vi "1_VNA_direct_spectrum_field_sweep_TEMPEATURE_(2D_PNA_m_Field_Direct_spec_RHUL).vi"() -> ()   [LabVIEW 2013]
uses:
  <vilib>/Analysis/baseanly.llb/Mean (DBL).vi
  <vilib>/Analysis/NI_AALBase.lvlib
panel:
  in  "Boolean 2":bool
  in  "?":enum32{"VNA"}(tab)
  out "Numeric":i32
  in  "Measurement \nper temperature":i32=3 caption="Delay Time (s)"
  out "Paused":bool
  in  "Boolean":bool
  in  "Delay Time (s)":dbl=3.0
  in  "?":enum32{"VNA"}(tab)
  in  "VNA Power dBm":dbl=-30.0 caption="VNA Power (dBm)" format="%#.3f"
  in  "Center Freq (Hz)":dbl=9000000000.0 caption="Center Freq (Hz):" format="%#.6p"
  in  "Span Freq:":dbl=14000000000.0 caption="Span Freq (Hz)" format="%#.3p"
  in  "Bandwidth:":dbl=10.0 caption="Bandwidth (1 to 1e6 Hz)" format="%#.3f"
  in  "Points:":i32=201 caption="Points"
  out "Phase (now)":dbl[](graph)
  out "Amplitude (now)":dbl[](graph)
  in  "Phase delay (ns)":dbl=53.6 format="%#_8g"
  in  "Offset (rad)":dbl
  out "Temperature sorted":dbl[](array[numeric])
  out "Phase Background Corrected":dbl[][](graph)
  out "Amplitude Background Corrected":dbl[][](graph)
  out "Phase Raw":dbl[][](graph)
  out "Amplitude Raw":dbl[][](graph)
  out "XY Graph":cluster{dbl[], dbl[]}(graph)
  out "Temp_start":dbl=2.0 format="%#_13g"
  out "Temp_end":dbl=16.0 format="%#_13g"
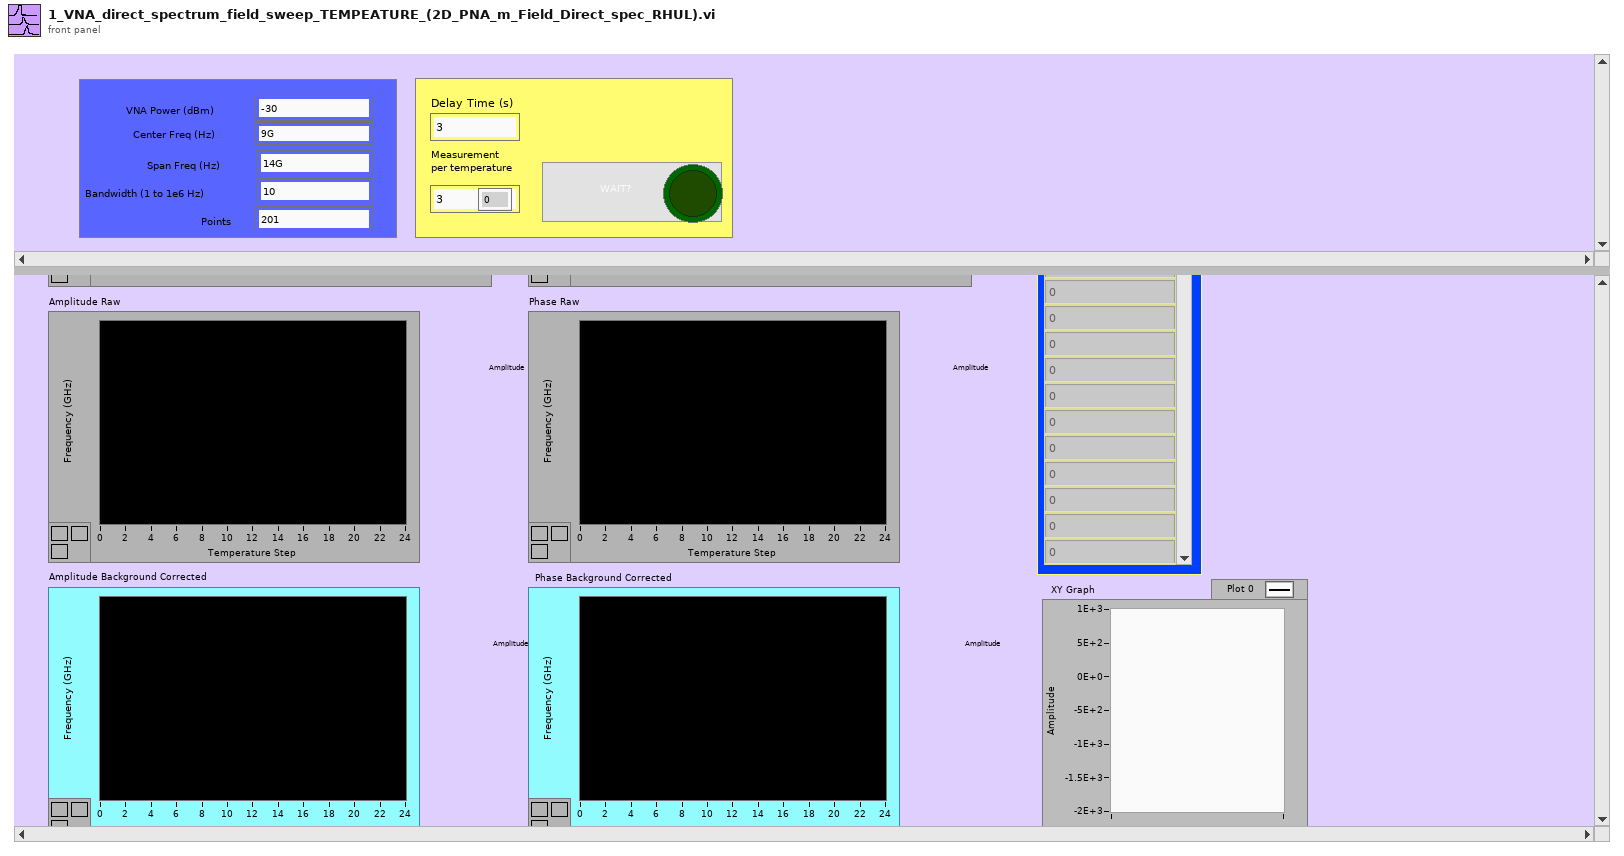
[diagram p1: front panel]
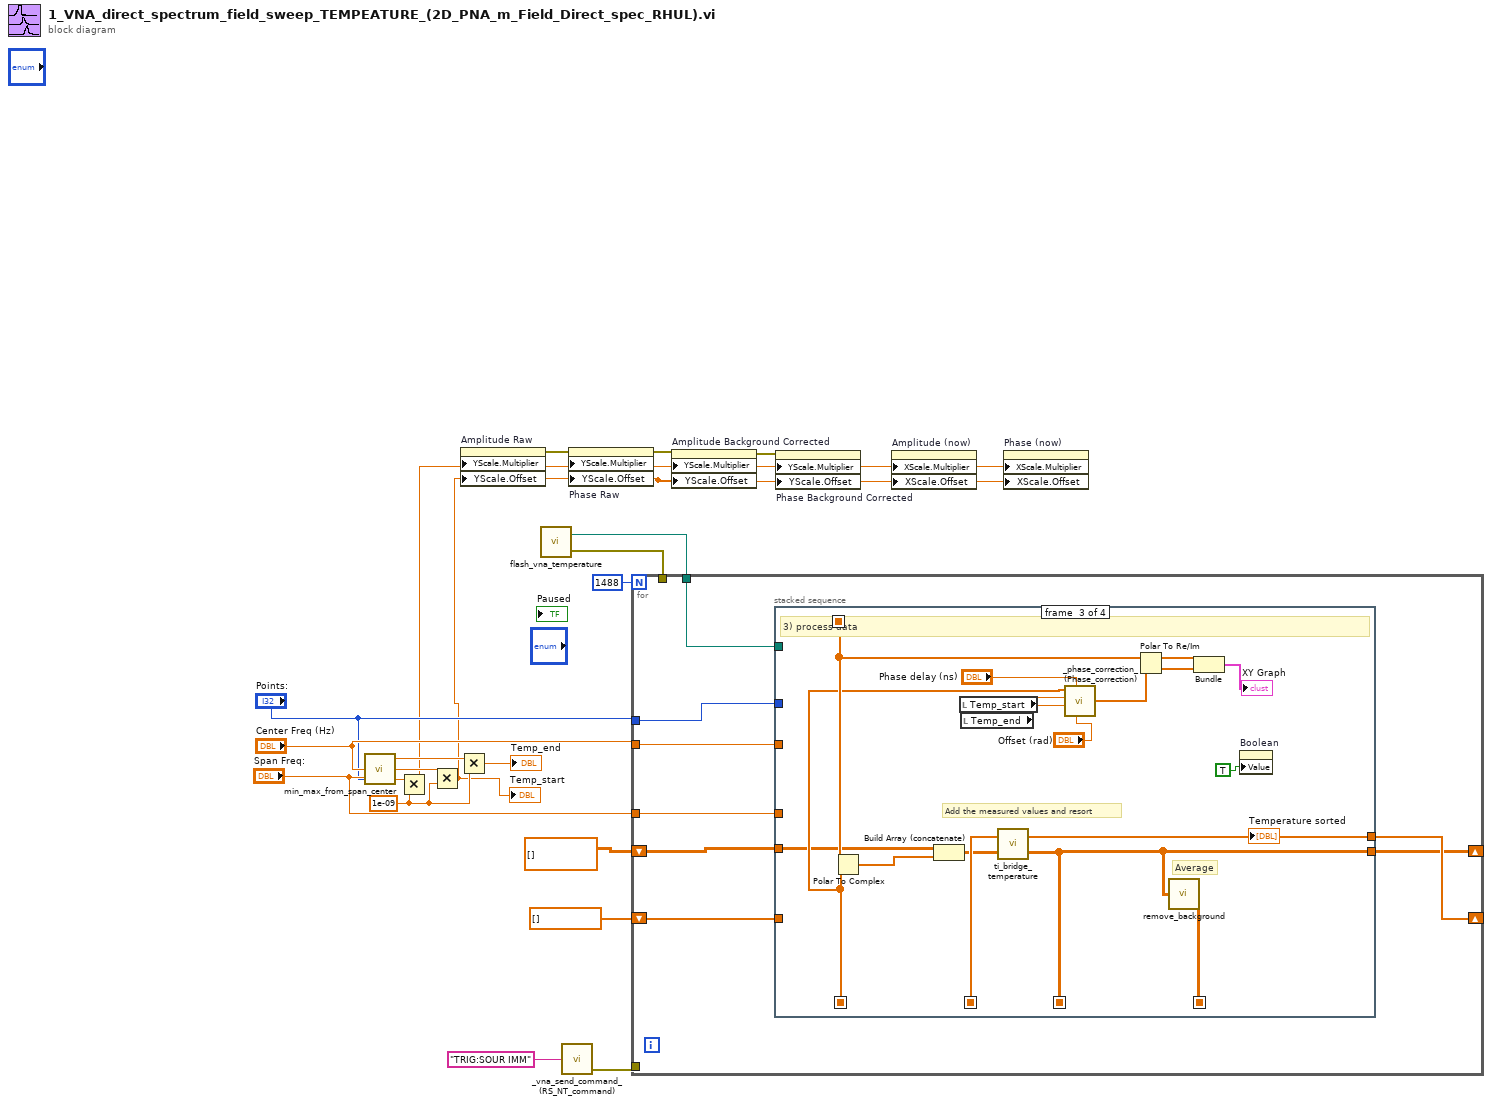
[diagram p0: block diagram]
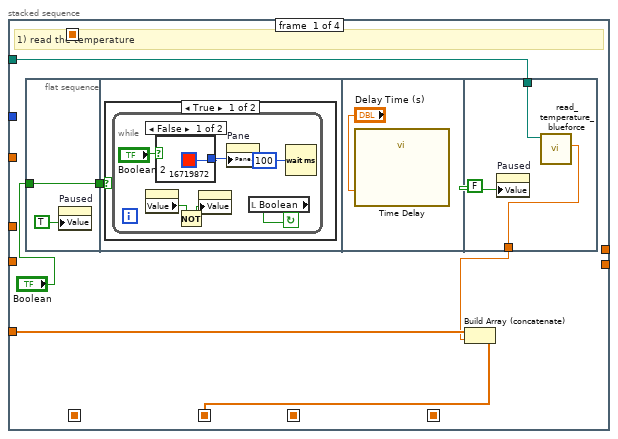
[diagram p2: hidden frame]
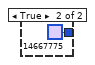
[diagram p3: hidden frame]
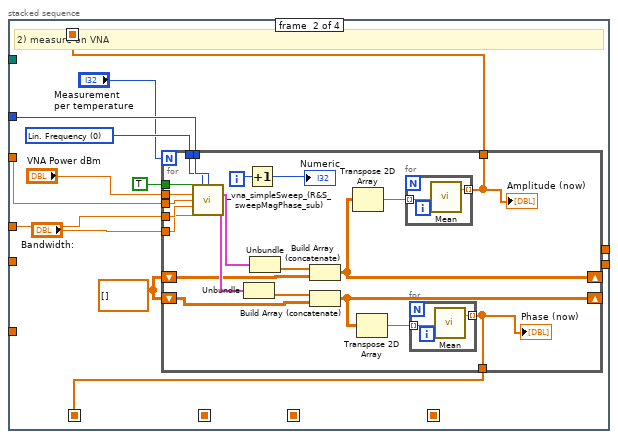
[diagram p5: hidden frame]
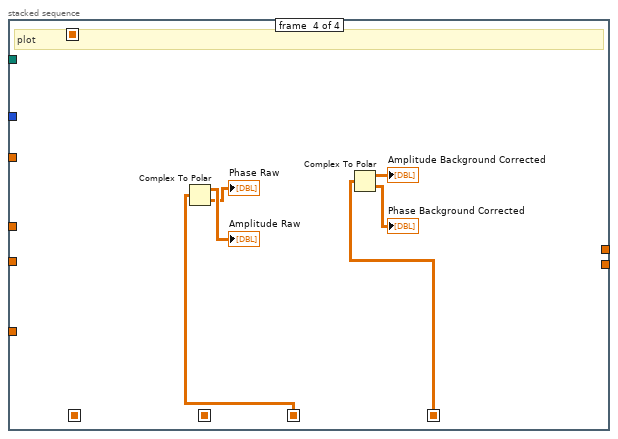
[diagram p6: hidden frame]
diagram:
  w13 = 1e-09
  n1 = call "min_max_from_span_center.vi"("No Points"="Points:", "Mid Point"="Center Freq (Hz)", "Span"="Span Freq:") -> ("Step"=w15:dbl, "Start"=w14:dbl, "End"=w18:dbl)
  n2 = Multiply(x=w15, y=w13) -> (x*y=w4:dbl)
  n3 = Multiply(x=w14, y=w13) -> (x*y=w3:dbl)
  "Temp_start" <- w3
  n4 = Multiply(x=w18, y=w13) -> (x*y=→"Temp_end":dbl)
  n5 = property on="Amplitude Raw" class="IntGraph (strict)"("YScale.Multiplier"=w4, "YScale.Offset"=w3) -> (error out=w7:errorcluster)  [unwired: 2 in, 1 out]
  n6 = call "flash_vna_temperature.vi"() -> ("error out"=w2:errorcluster, "File"=w1:path)  [unwired: 2 in]
  n7 = call "_vna_send_command_(RS_NT_command).vi"("Comand"="TRIG:SOUR IMM") -> ("error out"=w19:errorcluster)  [unwired: 4 in]
  n8 = property on="Phase Raw" class="IntGraph (strict)"(error in=w7, "YScale.Multiplier"=w4, "YScale.Offset"=w3) -> (error out=w5:errorcluster)  [unwired: 1 in, 1 out]
  n9 = for {
    N: 1488 -> [_]
    tunnel: "Center Freq (Hz)" -> [w28]
    tunnel: "Span Freq:" -> [w27]
    tunnel: "Points:" -> [w26]
    tunnel: w19 -> [_]
    shift-right: [w23] -> _
    shift-left: dbl[] [] -> [w25]
    shift-right: [w22] -> _
    shift-left: cdb[][] [] ("Array") -> [w24]
    tunnel: w2 -> [_]
    tunnel: w1 -> [w21]
    n10 = stacked-sequence {
      seq-local: [_ w52 _ _] -> [_ _ w99 _]
      seq-local: [_ w51 _ _] -> [_ _ w94 _]
      seq-local: [_ _ w86 _] -> [_ _ _ w107]
      seq-local: [w33 _ _ _] -> [_ _ w91 _]
      seq-local: [_ _ w87 _] -> [_ _ _ w106]
      tunnel: w28 -> [_ w54 _ _]
      tunnel: w27 -> [_ w59 _ _]
      tunnel: w26 -> [_ w60 _ _]
      tunnel: w25 -> [w34 _ _ _]
      tunnel: w24 -> [_ _ w93 _]
      tunnel: [_ _ w90 _] -> w23
      tunnel: [_ _ w87 _] -> w22
      tunnel: w21 -> [w29 _ _ _]
      frame #0 {
        # "1) read the temperature"
        n11 = flat-sequence {
          tunnel: "Boolean" -> [w36]
          tunnel: [w36] -> w31
          tunnel: w31 -> [w37]
          tunnel: [w48] -> w30
          tunnel: w29 -> [w47]
          frame #0 {
            n12 = property on="Paused" class="Bool (strict)"("Value"=TRUE ("Paused")) -> ()  [unwired: 2 in, 2 out]
          }
          frame #1 {
            n13 = case shown="True" w37 {
              frame True {
                n14 = while {
                  stop <- w43 continue-if-true
                  n15 = property on="Boolean 2" class="Bool (strict)"() -> ("Value"=w39:bool)  [unwired: 2 in, 2 out]
                  n16 = case shown="False" "Boolean 2" {
                    tunnel: [u32 16719872 u32 14667775] -> w42
                    frame False {
                    }
                    frame True {
                    }
                  }
                  n17 = Not(x=w39) -> (.not. x?=w38:bool)
                  n18 = property on="Boolean 2" class="Bool (strict)"("Value"=w38) -> ()  [unwired: 2 in, 2 out]
                  n19 = property on="Pane" class="Pane"("PaneColor"=w42) -> ()  [unwired: 2 in, 2 out]
                  n20 = local read "Boolean"() -> (w43:bool)
                  n21 = Wait (ms)(milliseconds to wait=u32 100) -> ()  [unwired: 1 out]
                }
              }
              frame False {
              }
            }
          }
          frame #2 {
            n22 = call "Time Delay"("Delay Time (s)"="Delay Time (s)") -> ()  [unwired: 10 in, 1 out]
          }
          frame #3 {
            n23 = property on="Paused" class="Bool (strict)"("Value"=FALSE ("Paused")) -> ()  [unwired: 2 in, 2 out]
            n24 = call "read_temperature_blueforce.vi"("file (use dialog)"=w47) -> ("MX Temperature"=w48:dbl)  [unwired: 9 in, 1 out]
          }
        }
        n25 = Build Array (concatenate)(w34, w30) -> (w33:dbl[])
      }
      frame #1 {
        w53 = dbl[][] []
        w58 = 0 items=["Lin. Frequency", "Log. Frequency", "Segmented Frequency", "Power", "Time", "CW Mode"] ("Sweep Type")
        # "2) measure on VNA"
        n26 = for {
          N: "Measurement \nper temperature" -> [_]
          tunnel: w60 -> [w79]
          tunnel: w59 -> [w78]
          tunnel: w58 -> [w77]
          tunnel: TRUE ("Boolean") -> [w76]
          tunnel: "VNA Power dBm" -> [w75]
          tunnel: "Bandwidth:" -> [w74]
          tunnel: w54 -> [w73]
          shift-right: [w68] -> _
          shift-left: w53 -> [w70]
          shift-right: [w65] -> _
          shift-left: w53 -> [w69]
          tunnel: [w64] -> w52
          tunnel: [w63] -> w51
          i -> [w62]
          n27 = call "_vna_simpleSweep_(R&S_sweepMagPhase_sub).vi"("Boolean"=w76, "Sweep Type"=w77, "Points:"=w79, "Power dBm"=w75, "Center Freq:"=w73, "Span Freq:"=w78, "Bandwidth:"=w74) -> ("Lin Mag"=w81:cluster{dbl[], dbl[]}, "Phase"=w80:cluster{dbl[], dbl[]})  [unwired: 7 in]
          n28 = Unbundle(w80) -> (w72:dbl[])  [unwired: 1 out]
          n29 = Increment(x=w62) -> (x+1=→"Numeric":i32)
          n30 = Unbundle(w81) -> (w71:dbl[])  [unwired: 1 out]
          n31 = Build Array (concatenate)(w71, w70) -> (w68:dbl[][])
          n32 = Build Array (concatenate)(w72, w69) -> (w65:dbl[][])
          n33 = Transpose 2D Array(2D array=w68) -> (transposed array=w67:dbl[][])
          n34 = Transpose 2D Array(2D array=w65) -> (transposed array=w66:dbl[][])
          n35 = for {
            tunnel: w67 -> [w85] mode=indexing
            tunnel: [w84] -> w64 mode=indexing
            n36 = call-poly <vilib>:"Mean.vi"("X"=w85) -> ("mean"=w84:dbl)  [unwired: 1 out]
          }
          "Amplitude (now)" <- w64
          n37 = for {
            tunnel: w66 -> [w83] mode=indexing
            tunnel: [w82] -> w63 mode=indexing
            n38 = call-poly <vilib>:"Mean.vi"("X"=w83) -> ("mean"=w82:dbl)  [unwired: 1 out]
          }
          "Phase (now)" <- w63
        }
      }
      frame #2 {
        # "Average"
        # "Add the measured values and resort"
        # "3) process data"
        n39 = Polar To Complex(1:w94, 2:w99) -> (0:w92:cdb[])
        n40 = Build Array (concatenate)(w93, w92) -> (w88:cdb[][])
        n41 = local read "Temp_start"() -> (w96:dbl)
        n42 = local read "Temp_end"() -> (w97:dbl)
        n43 = call "ti_bridge_temperature.vi"("Z"=w88, "Temperature"=w91) -> ("Z_array sorted"=w87:cdb[][], "Temperature sorted"=w90:dbl[])
        "Temperature sorted" <- w90
        n44 = call "_phase_correction_(Phase_correction).vi"("offset"="Offset (rad)", "Delay (ns)"="Phase delay (ns)", "f1 (GHz)"=w97, "f0 (GHz)"=w96, "Phase in"=w94) -> ("Phase out"=w100:dbl[])  [unwired: 4 in]
        n45 = Polar To Re/Im(2:w100, 3:w99) -> (0:w102:dbl[], 1:w103:dbl[])
        n46 = call "remove_background.vi"("Array in"=w87) -> ("Array out"=w86:cdb[][])  [unwired: 1 in]
        n47 = Bundle(w103, w102) -> (→"XY Graph":cluster{dbl[], dbl[]})  [unwired: 1 in]
        n48 = property on="Boolean" class="Bool (strict)"("Value"=TRUE ("Paused")) -> ()  [unwired: 2 in, 2 out]
      }
      frame #3 {
        # "plot"
        n49 = Complex To Polar(r * e^(i*theta)=w106) -> (r=→"Amplitude Raw":dbl[][], theta=→"Phase Raw":dbl[][])
        n50 = Complex To Polar(r * e^(i*theta)=w107) -> (r=→"Amplitude Background Corrected":dbl[][], theta=→"Phase Background Corrected":dbl[][])
      }
    }
  }
  n51 = property on="Amplitude Background Corrected" class="IntGraph (strict)"(error in=w5, "YScale.Multiplier"=w4, "YScale.Offset"=w3) -> (error out=w6:errorcluster)  [unwired: 1 in, 1 out]
  n52 = property on="Phase Background Corrected" class="IntGraph (strict)"(error in=w6, "YScale.Multiplier"=w4, "YScale.Offset"=w3) -> ()  [unwired: 1 in, 2 out]
  n53 = property on="Amplitude (now)" class="WFGraph (strict)"("XScale.Multiplier"=w4, "XScale.Offset"=w3) -> ()  [unwired: 2 in, 2 out]
  n54 = property on="Phase (now)" class="WFGraph (strict)"("XScale.Multiplier"=w4, "XScale.Offset"=w3) -> ()  [unwired: 2 in, 2 out]
